vi "Test.vi"() -> ()   [LabVIEW 2024]
uses:
  <vilib>/vision/NI_Vision_Development_Module.lvlib
  <vilib>/Utility/config.llb/NI_LVConfig.lvlib
  <vilib>/Utility/config.llb/Read Key (I32).vi
  <vilib>/Utility/config.llb/Read Key (Double).vi
  <vilib>/Utility/config.llb/Read Key (Boolean).vi
panel:
  in  "Stop Button":bool
  in  "Boolean":bool
  in  "Numeric":dbl
  out "Cluster 2":cluster{"Numeric":dbl, "Boolean":bool}
  out "Cluster":cluster{"Numeric":dbl, "Boolean":bool}
  out "element 3":i32
  out "element 2":i32
  out "element":i32
  in  "Muster speichern?":bool
  out "Nicht vorhandene Konfigs (werden erstellt haben aber größe 0 KB)":string[](array[string])
  out "error out":errorcluster
  out "ISO":T1(plugin-control)
  # "0,64"
  # "1,12"
  # "0,35"
  # "0,75"
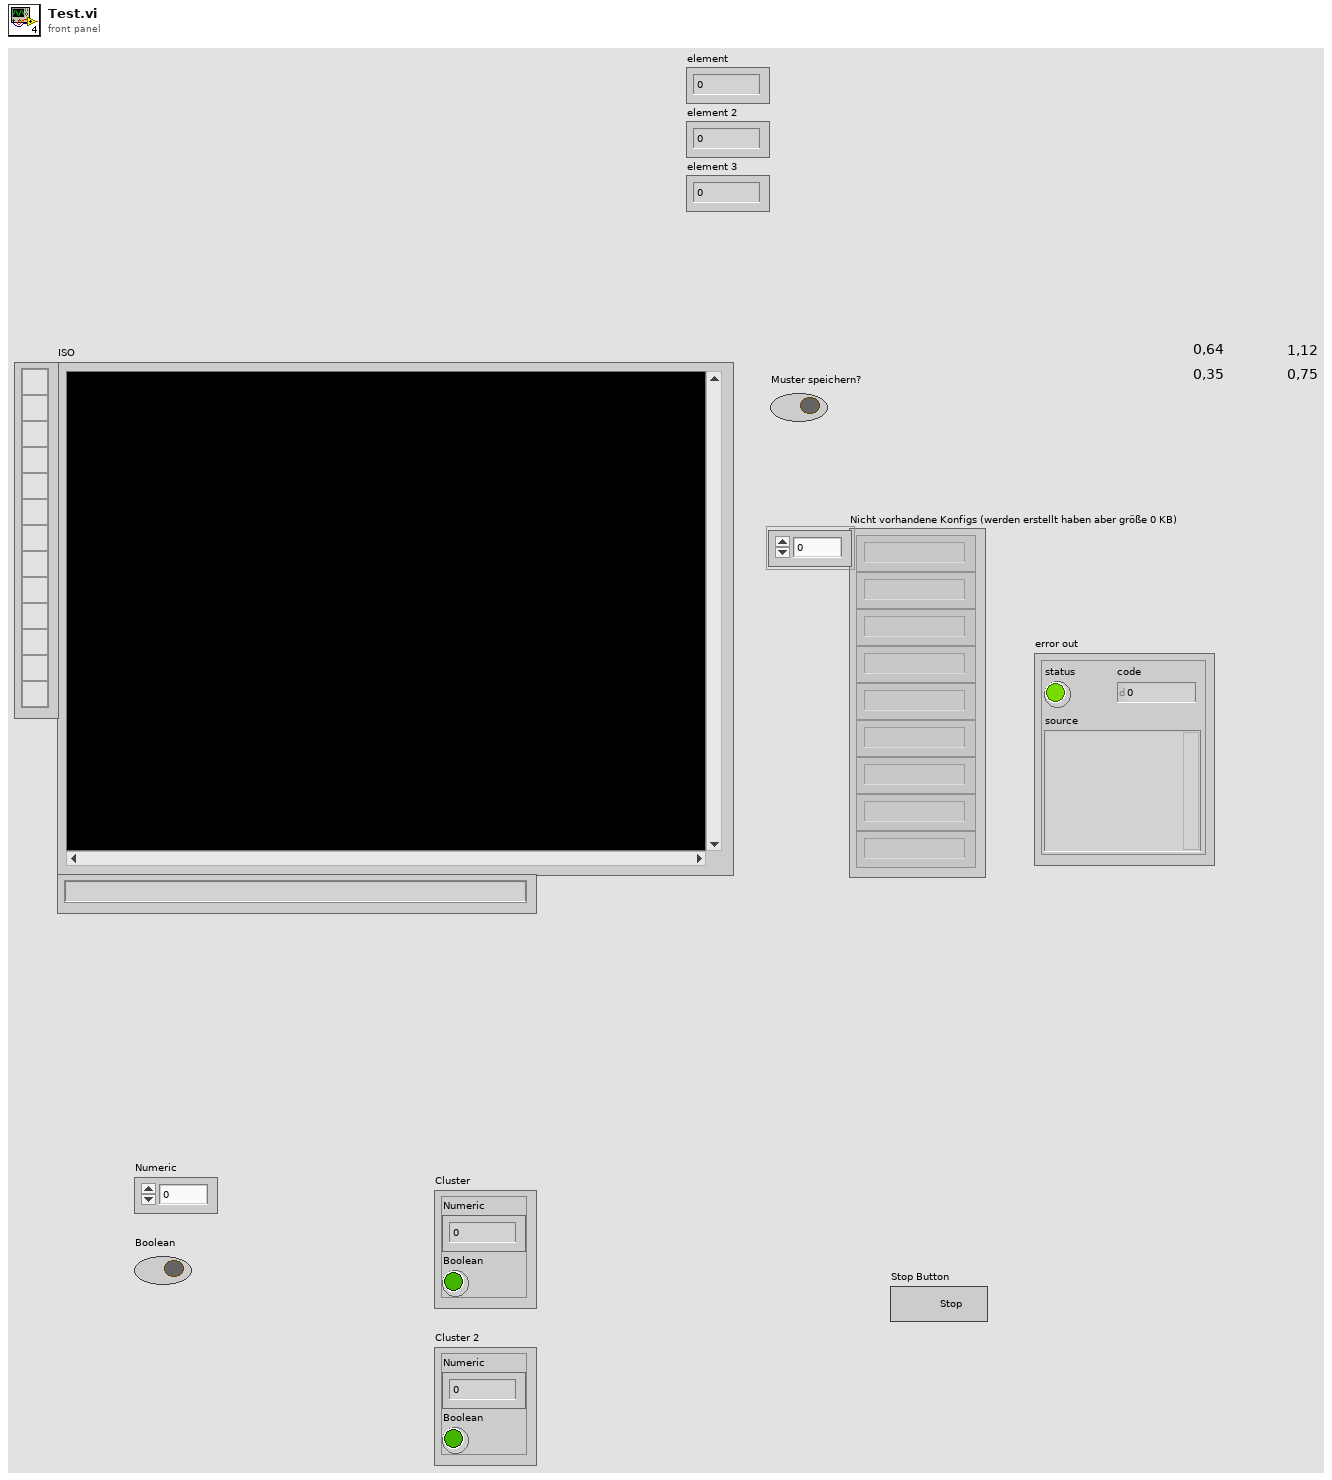
[diagram p1: front panel]
types:
  T1 = typedef "IMAQ Image.ctl" = refnum<image>
  T2 = typedef "IMAQ Rectangle" = cluster{"Left":i32, "Top":i32, "Right":i32, "Bottom":i32, "Rotation":dbl}
  T3 = typedef "NI_LVConfig.lvlib/Config Data RefNum.ctl" = refnum<k1>
  T4 = cluster{"Object Center":cluster{"X":sgl, "Y":sgl}, "Bounding Box":cluster{"X Left":i32, "Y Top":i32, "X Right":i32, "Y Bottom":i32}, "Area":sgl, "Orientation":sgl, "Aspect Ratio":sgl, "Nb Holes":i32}[]
  T5 = typedef "ROI Descriptor" = cluster{"Global Rectangle":i32[], "Contours":cluster{"ID":enum32{"External", "Internal"}, "Type":u32, "Coordinates":i32[]}[]}
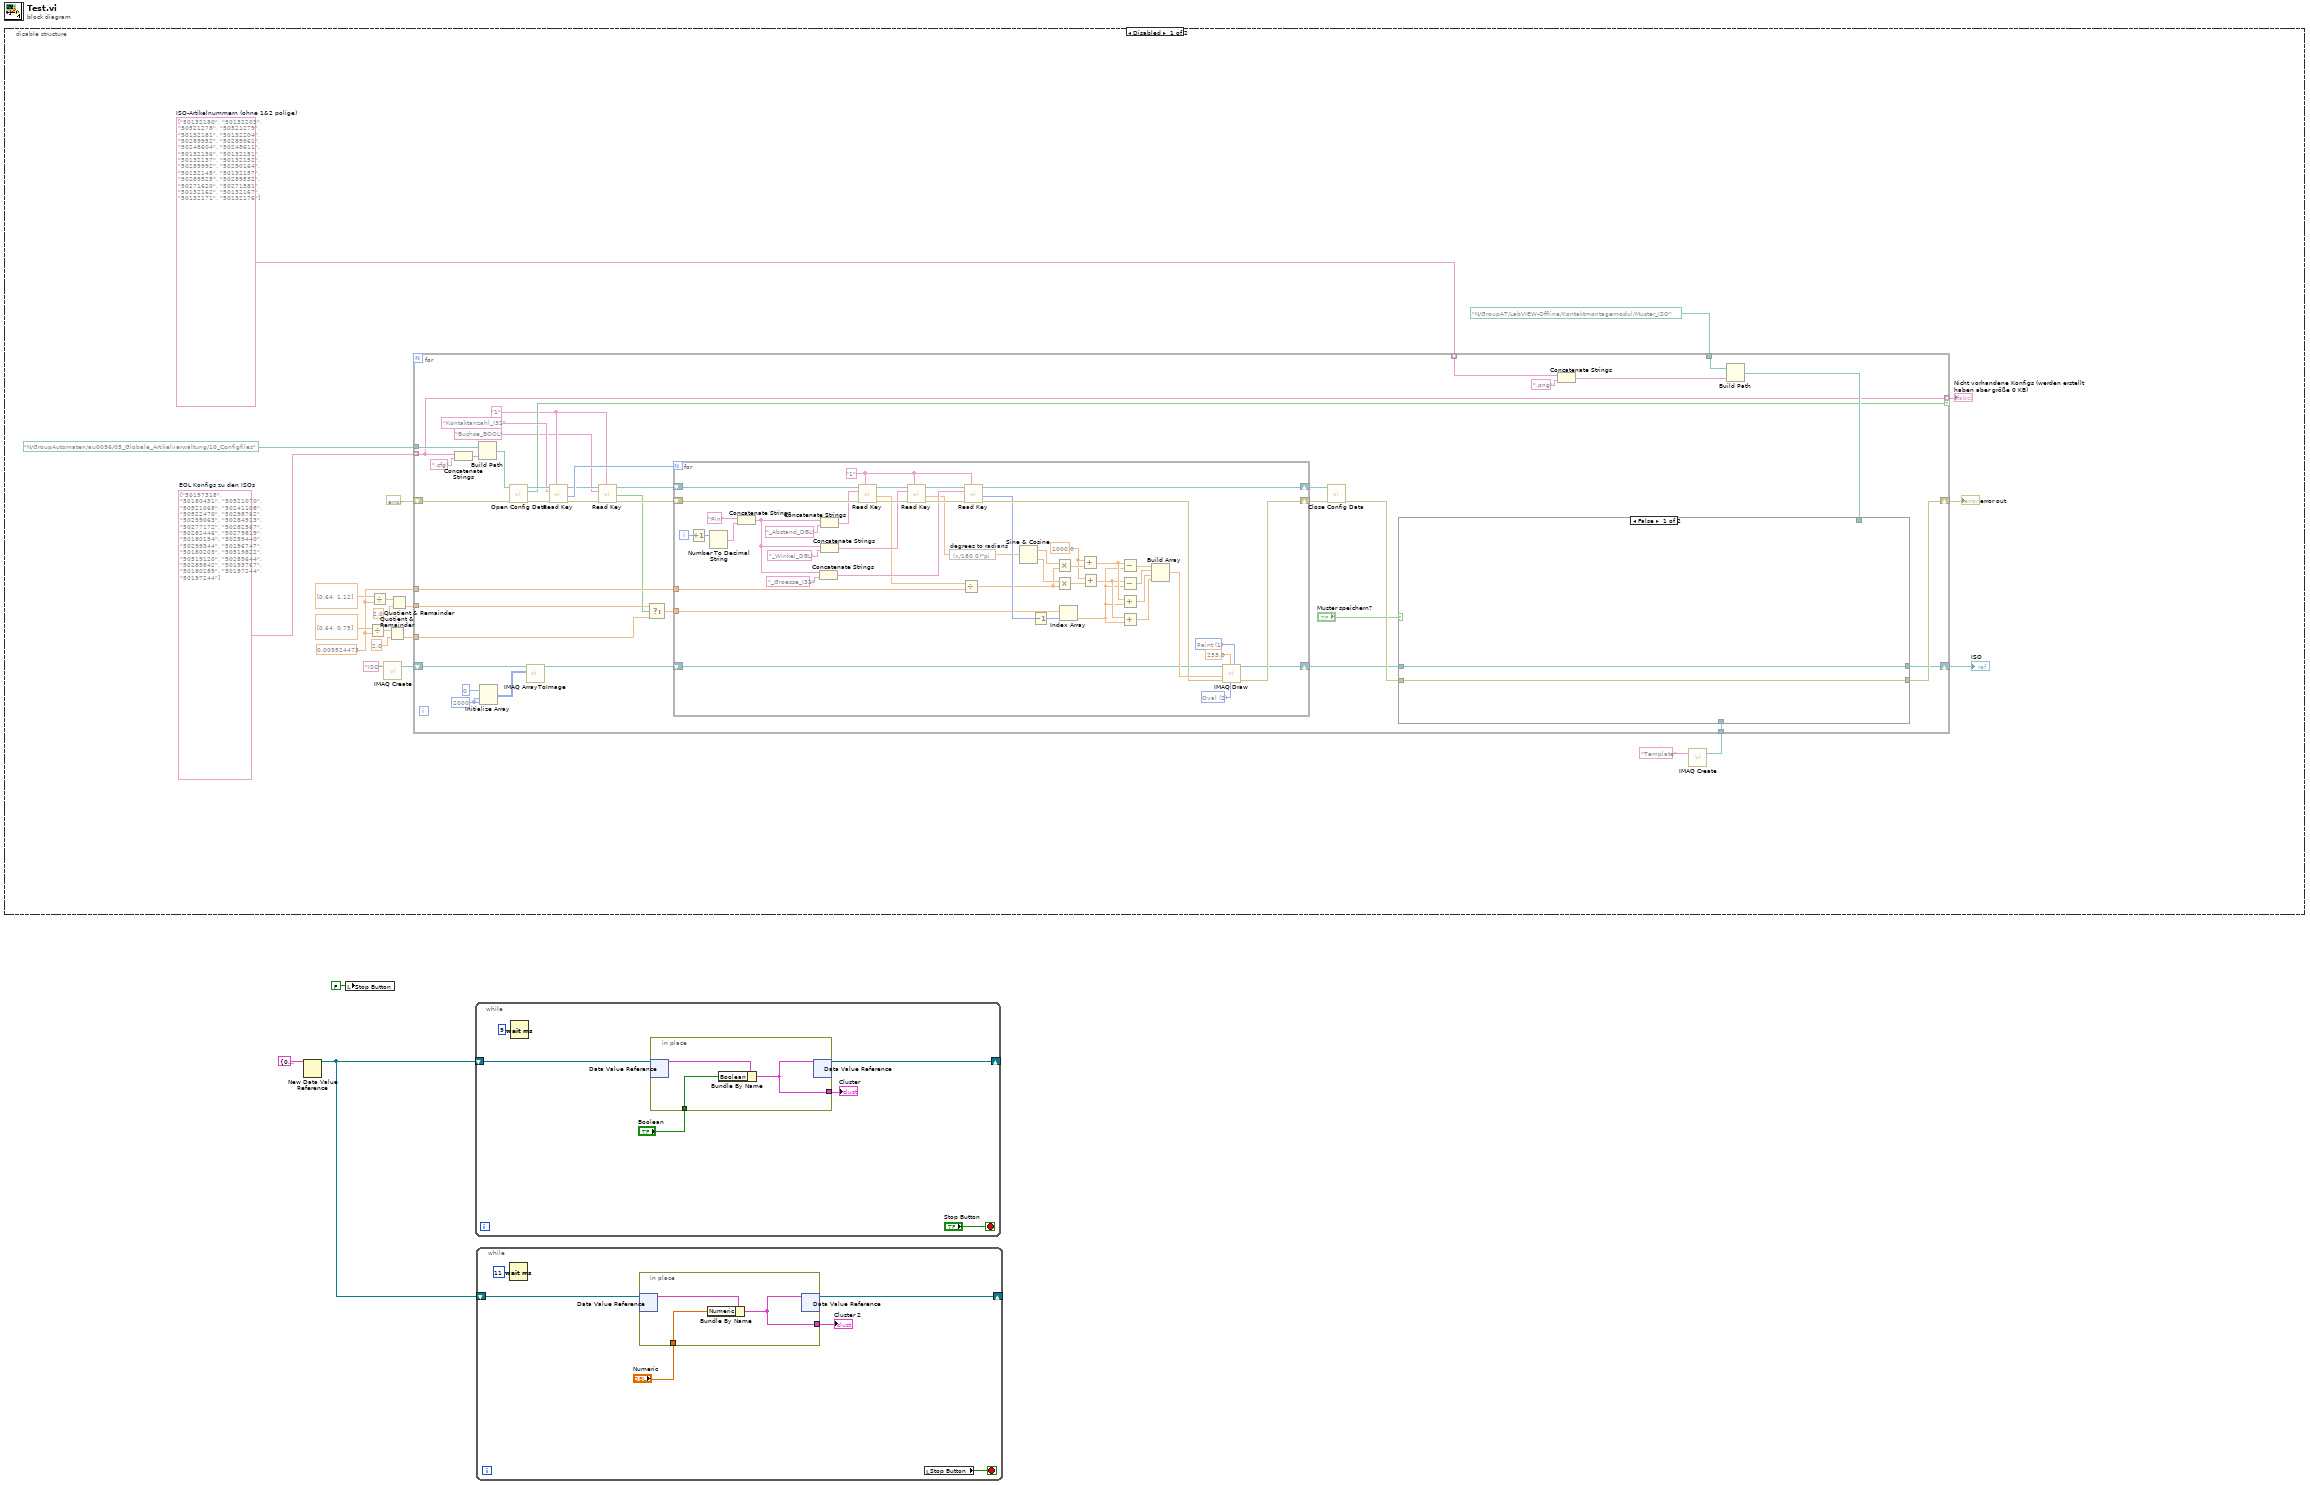
[diagram p0: block diagram]
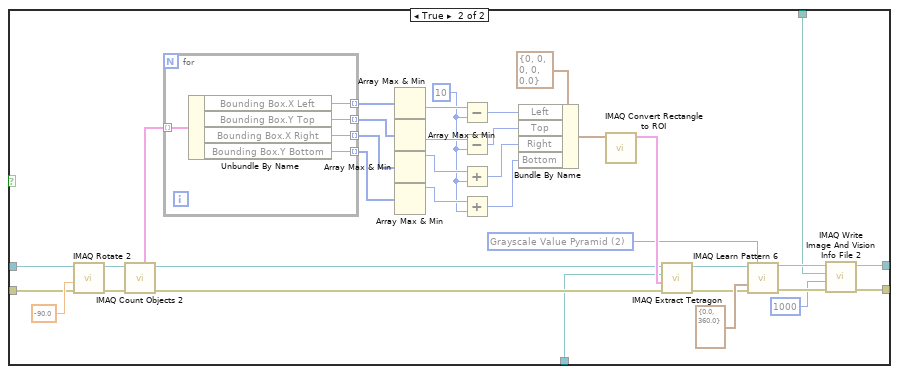
[diagram p2: hidden frame]
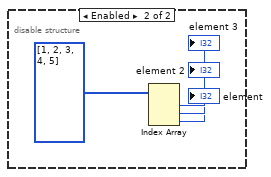
[diagram p3: hidden frame]
diagram:
  n1 = disable-structure shown="Disabled" {
    frame Disabled {
      w4 = string[] ["50132180", "50132203", "50521278", "50521279", "50132181", "50132204", "50289952", "50289961", "50248604", "50248611", "50132136", "50132151", "50132137", "50132152", "50289992", "50290164", "50132145", "50132157", "50289525", "50289532", "50271620", "50271581", "50132162", "50132167", "50132171", "50132176"]  # ISO-Artikelnummern (ohne 1&2 polige)
      w5 = string[] ["50197318", "50180431", "50521070", "50521068", "50241108", "50522470", "50298762", "50299063", "50284913", "50277172", "50282567", "50282446", "50279819", "50180194", "50299440", "50299344", "50196747", "50180203", "50519822", "50519120", "50289644", "50289842", "50193767", "50180289", "50197244", "50197244"]  # EOL Konfigs zu den ISOs
      w7 = 0.009524473
      n2 = Divide(x=dbl[] [0.64, 0.75] ("Kontaktgrößen"), y=w7) -> (x/y=w10:dbl[])
      n3 = Divide(x=dbl[] [0.64, 1.12] ("Kontaktgrößen"), y=w7) -> (x/y=w22:dbl[])
      n4 = call "IMAQ Create"("Image Name"="ISO") -> ("New Image"=w13:T1)  [unwired: 4 in, 1 out]
      n5 = Quotient & Remainder(x=w10, y=2.0) -> (floor(x/y)=w6:dbl[])  [unwired: 1 out]
      n6 = Quotient & Remainder(x=w22, y=2.0) -> (floor(x/y)=w21:dbl[])  [unwired: 1 out]
      n7 = call "IMAQ Create"("Image Name"="Template") -> ("New Image"=w17:T1)  [unwired: 4 in, 1 out]
      n8 = for {
        tunnel: path "N:/GroupAutomaten/au0096/05_Globale_Artikelverwaltung/10_Configfiles" ("Folder Path") -> [w64]
        tunnel: w21 -> [w28]
        tunnel: w7 -> [w54]
        tunnel: w5 -> [w45] mode=indexing
        shift-right: [w51] -> w19
        shift-left: errorcluster {"status"=FALSE, "code"=0, "source"=""} ("error in (no error)") -> [w53]
        tunnel: w17 -> [w52]
        tunnel: path "N:/GroupAT/LabVIEW-Offline/Kontaktmontagemodul/Muster_ISO" ("File Path") -> [w48]
        tunnel: w4 -> [w46] mode=indexing
        tunnel: [w45] -> w15 mode=indexing if=w44
        shift-right: [w38] -> w12
        shift-left: w13 -> [w40]
        tunnel: w6 -> [w26]
        w41 = 2000 ("dimension size")
        w31 = "1" ("section")
        n9 = Concatenate Strings(w45, ".cfg" ("string")) -> (w62:string)
        n10 = Build Path(base path=w64, name or relative path=w62) -> (appended path=w61:path)
        n11 = Initialize Array(u8 0, w41, w41) -> (w43:u8[][])
        n12 = call <vilib>:"Open Config Data.vi"("error in (no error)"=w53, "configuration file path"=w61) -> ("error out"=w59:errorcluster, "file created?"=w44:bool, "refnum"=w60:T3)  [unwired: 7 in]
        n13 = call "IMAQ ArrayToImage"("Image Pixels (U8)"=w43, "Image"=w40) -> ("Image Out"=w39:T1)  [unwired: 8 in, 1 out]
        n14 = call-poly <vilib>:"Read Key.vi"("section"=w31, "error in (no error)"=w59, "key"="Kontaktanzahl_I32", "refnum"=w60) -> ("error out"=w34:errorcluster, "value"=w55:i32, "refnum out"=w35:T3)  [unwired: 4 in, 1 out]
        n15 = call-poly <vilib>:"Read Key.vi"("section"=w31, "error in (no error)"=w34, "key"="Buchse_BOOL", "refnum"=w35) -> ("error out"=w33:errorcluster, "value"=w29:bool, "refnum out"=w32:T3)  [unwired: 4 in, 1 out]
        n16 = Select(t=w28, s=w29, f=w26) -> (s? t:f=w27:dbl[])
        n17 = for {
          N: w55 -> [_]
          shift-right: [w119] -> w57
          shift-left: w33 -> [w152]
          shift-right: [w122] -> w56
          shift-left: w32 -> [w153]
          shift-right: [w117] -> w36
          shift-left: w39 -> [w118]
          tunnel: w27 -> [w114]
          tunnel: w54 -> [w111]
          i -> [w151]
          w130 = 1000.0
          w140 = u16 1 items=["Frame", "Paint", "Invert Frame", "Invert Paint"] ("Draw Mode")
          w139 = u16 2 items=["Line", "Rectangle", "Oval"] ("Shape to draw")
          w112 = "1" ("section")
          n18 = Increment(x=w151) -> (x+1=w149:i32)
          n19 = Number To Decimal String(number=w149) -> (decimal integer string=w148:string)  [unwired: 1 in]
          n20 = Concatenate Strings("Pin", w148) -> (w126:string)
          n21 = Concatenate Strings(w126, "_Groesse_I32" ("key")) -> (w121:string)
          n22 = Concatenate Strings(w126, "_Abstand_DBL" ("key")) -> (w146:string)
          n23 = Concatenate Strings(w126, "_Winkel_DBL" ("key")) -> (w142:string)
          n24 = call-poly <vilib>:"Read Key.vi"("section"=w112, "error in (no error)"=w152, "key"=w146, "refnum"=w153) -> ("error out"=w144:errorcluster, "value"=w109:dbl, "refnum out"=w145:T3)  [unwired: 4 in, 1 out]
          n25 = call-poly <vilib>:"Read Key.vi"("section"=w112, "error in (no error)"=w144, "key"=w142, "refnum"=w145) -> ("error out"=w123:errorcluster, "value"=w108:dbl, "refnum out"=w124:T3)  [unwired: 4 in, 1 out]
          n26 = expression code="(x/180.0)*pi" "degrees to radians"(w108) -> (w107:dbl)
          n27 = Divide(x=w109, y=w111) -> (x/y=w110:dbl)
          n28 = call-poly <vilib>:"Read Key.vi"("section"=w112, "error in (no error)"=w123, "key"=w121, "refnum"=w124) -> ("error out"=w120:errorcluster, "value"=w116:i32, "refnum out"=w122:T3)  [unwired: 4 in, 1 out]
          n29 = Sine & Cosine(0:w107) -> (1:w138:dbl, 2:w137:dbl)
          n30 = Decrement(x=w116) -> (x-1=w115:i32)
          n31 = Multiply(x=w138, y=w110) -> (x*y=w132:dbl)
          n32 = Multiply(x=w137, y=w110) -> (x*y=w129:dbl)
          n33 = Index Array(array=w114, index=w115) -> (element=w113:dbl)
          n34 = Add(x=w130, y=w132) -> (x+y=w131:dbl)
          n35 = Add(x=w130, y=w129) -> (x+y=w128:dbl)
          n36 = Subtract(x=w131, y=w113) -> (x-y=w136:dbl)
          n37 = Subtract(x=w128, y=w113) -> (x-y=w135:dbl)
          n38 = Add(x=w131, y=w113) -> (x+y=w134:dbl)
          n39 = Add(x=w128, y=w113) -> (x+y=w133:dbl)
          n40 = Build Array(w136, w135, w134, w133) -> (w127:dbl[])
          n41 = call "IMAQ Draw"("Draw Mode"=w140, "Shape to draw"=w139, "Pixel Color"=sgl 255.0, "error in (no error)"=w120, "Coordinates"=w127, "Image Src"=w118) -> ("error out"=w119:errorcluster, "Image Dst Out"=w117:T1)  [unwired: 4 in]
        }
        n42 = call <vilib>:"Close Config Data.vi"("error in (no error)"=w57, "refnum"=w56) -> ("error out"=w37:errorcluster)  [unwired: 8 in, 1 out]
        n43 = Concatenate Strings(w46, ".png" ("string")) -> (w49:string)
        n44 = Build Path(base path=w48, name or relative path=w49) -> (appended path=w47:path)
        n45 = case shown="False" "Muster speichern?" {
          tunnel: w52 -> [_ w77]
          tunnel: [w65 w76] -> w51
          tunnel: w47 -> [_ w75]
          tunnel: [w66 w73] -> w38
          tunnel: w37 -> [w65 w69]
          tunnel: w36 -> [w66 w68]
          frame False {
          }
          frame True {
            w81 = 10 ("y")
            w96 = 2 items=["All", "Low Discrepancy Sampling", "Grayscale Value Pyramid", "Gradients Pyramid"] ("Algorithm")
            n46 = call "IMAQ Rotate 2"("error in (no error)"=w69, "Angle (degrees)"=-90.0, "Image Src"=w68) -> ("error out"=w70:errorcluster, "Image Dst Out"=w67:T1)  [unwired: 7 in]
            n47 = call "IMAQ Count Objects 2"("error in (no error)"=w70, "Image"=w67) -> ("error out"=w95:errorcluster, "Image Out"=w94:T1, "Objects"=w93:T4)  [unwired: 5 in, 2 out]
            n48 = for {
              tunnel: w93 -> [w106] mode=indexing
              tunnel: [w105] -> w92 mode=indexing
              tunnel: [w104] -> w87 mode=indexing
              tunnel: [w103] -> w84 mode=indexing
              tunnel: [w102] -> w83 mode=indexing
              n49 = Unbundle By Name(w106) -> ("Bounding Box.X Left"=w105:i32, "Bounding Box.Y Top"=w104:i32, "Bounding Box.X Right"=w103:i32, "Bounding Box.Y Bottom"=w102:i32)
            }
            n50 = Array Max & Min(array=w92) -> (min value=w91:i32)  [unwired: 3 out]
            n51 = Array Max & Min(array=w87) -> (min value=w88:i32)  [unwired: 3 out]
            n52 = Array Max & Min(array=w84) -> (max value=w85:i32)  [unwired: 3 out]
            n53 = Array Max & Min(array=w83) -> (max value=w82:i32)  [unwired: 3 out]
            n54 = Subtract(x=w91, y=w81) -> (x-y=w89:i32)
            n55 = Subtract(x=w88, y=w81) -> (x-y=w86:i32)
            n56 = Add(x=w85, y=w81) -> (x+y=w80:i32)
            n57 = Add(x=w82, y=w81) -> (x+y=w79:i32)
            n58 = Bundle By Name(cluster=T2 {"Left"=0, "Top"=0, "Right"=0, "Bottom"=0, "Rotation"=0.0} ("Rectangle"), "Left"=w89, "Top"=w86, "Right"=w80, "Bottom"=w79) -> (w78:T2)
            n59 = call "IMAQ Convert Rectangle to ROI"("Rectangle"=w78) -> ("ROI Descriptor"=w98:T5)  [unwired: 8 in, 1 out]
            n60 = call-poly "IMAQ Extract Tetragon"("error in (no error)"=w95, "ROI Descriptor"=w98, "Image Dst"=w77, "Image Src"=w94) -> ("error out"=w71:errorcluster, "Image Dst Out"=w72:T1)  [unwired: 6 in]
            n61 = call "IMAQ Learn Pattern 6"("Image"=w72, "Algorithm"=w96, "Angle Range"=cluster{"Start Angle":sgl, "End Angle":sgl} {"Start Angle"=0.0, "End Angle"=360.0}, "error in (no error)"=w71) -> ("Template Image Out"=w101:T1, "error out"=w100:errorcluster)  [unwired: 9 in, 1 out]
            n62 = call "IMAQ Write Image And Vision Info File 2"("error in (no error)"=w100, "Image Quality"=u32 1000, "File Path"=w75, "Image"=w101) -> ("error out"=w76:errorcluster, "Image Out (duplicate)"=w73:T1)  [unwired: 6 in]
          }
        }
      }
      "ISO" <- w12
      "error out" <- w19
      "Nicht vorhandene Konfigs (werden erstellt haben aber größe 0 KB)" <- w15
    }
    frame Enabled {
      n63 = Index Array(array=i32[] [1, 2, 3, 4, 5]) -> (element #1=→"element":i32, element #2=→"element 2":i32, element #3=→"element 3":i32)  [unwired: 3 in]
    }
  }
  n64 = New Data Value Reference(data value=cluster{"Numeric":dbl, "Boolean":bool} {"Numeric"=0.0, "Boolean"=FALSE} ("output cluster")) -> (data value reference=w1:refnum<data-value>)  [unwired: 1 in, 1 out]
  n65 = local write "Stop Button"(FALSE ("Stop Button")) -> ()
  n66 = while {
    shift-right: [w159] -> _
    shift-left: w1 -> [w161]
    stop <- "Stop Button" stop-if-true
    n67 = Wait (ms)(milliseconds to wait=u32 9) -> ()  [unwired: 1 out]
    n68 = in-place {
      in-place-border: "Boolean" -> [w165]
      in-place-border: [w164] -> w158
      n69 = in-place-dvr #1(w161) -> (w166:cluster{"Numeric":dbl, "Boolean":bool})  [unwired: 1 out]
      n70 = Bundle By Name(cluster=w166, "Boolean"=w165) -> (w164:cluster{"Numeric":dbl, "Boolean":bool})
      n71 = in-place-dvr #1(w164) -> (w159:refnum<data-value>)  [unwired: 1 out]
    }
    "Cluster" <- w158
  }
  n72 = while {
    shift-right: [w169] -> _
    shift-left: w1 -> [w170]
    stop <- w172 stop-if-true
    n73 = Wait (ms)(milliseconds to wait=u32 11) -> ()  [unwired: 1 out]
    n74 = in-place {
      in-place-border: "Numeric" -> [w174]
      in-place-border: [w173] -> w167
      n75 = in-place-dvr #2(w170) -> (w175:cluster{"Numeric":dbl, "Boolean":bool})  [unwired: 1 out]
      n76 = Bundle By Name(cluster=w175, "Numeric"=w174) -> (w173:cluster{"Numeric":dbl, "Boolean":bool})
      n77 = in-place-dvr #2(w173) -> (w169:refnum<data-value>)  [unwired: 1 out]
    }
    "Cluster 2" <- w167
    n78 = local read "Stop Button"() -> (w172:bool)
  }
